vi "save_temperature_and_pressure_to_excel.vi"() -> ()   [LabVIEW 2019]
uses:
  <vilib>/Utility/NIReport.llb/Report Type.ctl
  <vilib>/Utility/NIReport.llb/Append Text Table to Report (wrap).vi
  <vilib>/Utility/NIReport.llb/NI_report.lvclass
  <vilib>/Utility/NIReport.llb/NI_ReportGenerationCore.lvlib
  <vilib>/Utility/NIReport.llb/Excel/NI_Excel.lvclass
panel:
  in  "report file path":path
  in  "stop":bool
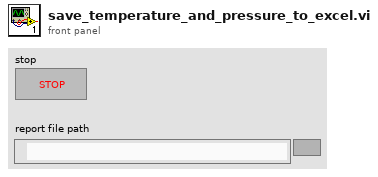
[diagram p1: front panel]
types:
  T1 = typedef "NI_ReportGenerationCore.lvlib/Report Type.ctl" = enum16{"HTML", "Word", "Excel"}
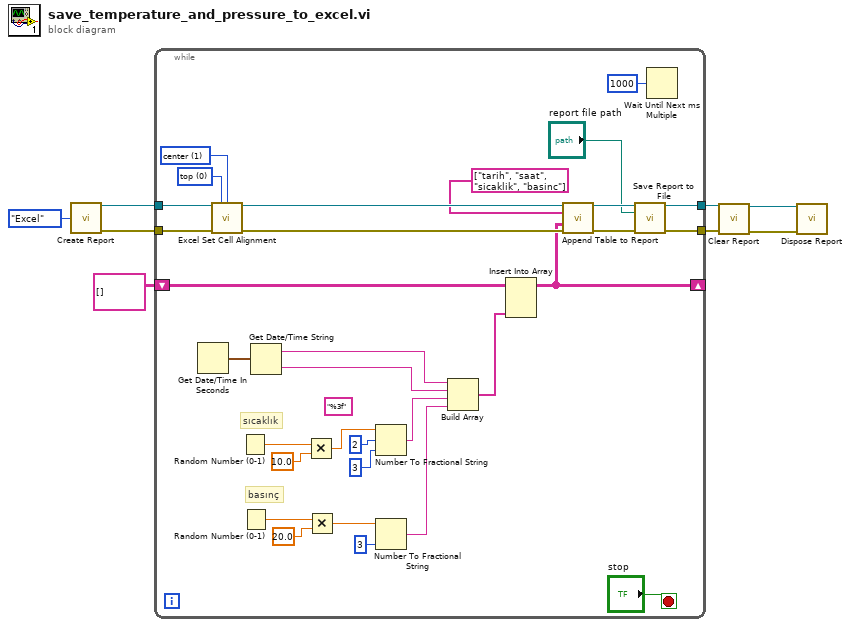
[diagram p0: block diagram]
diagram:
  n1 = call <vilib>:"Create Report.vi"("report type"=Report_Type."Excel") -> ("report out"=w7:refnum<class "NI_report.lvclass">, "error out"=w6:errorcluster)  [unwired: 13 in]
  n2 = while {
    tunnel: w7 -> [w35]
    tunnel: w6 -> [w34]
    tunnel: [w31] -> w4
    tunnel: [w30] -> w3
    shift-right: [w19] -> _
    shift-left: string[][] [] -> [w24]
    stop <- "stop" stop-if-true
    (unwired) "%3f" ("format string")
    w32 = 1 items=["left", "center", "right"] ("horizontal alignment (left)")
    w33 = 0 items=["top", "center", "bottom"] ("vertical alignment (top)")
    # "basınç"
    # "sıcaklık"
    n3 = Get Date/Time In Seconds() -> (seconds since 1Jan1904=w29:timestamp)
    n4 = call <vilib>:"Excel Set Cell Alignment.vi"("report in"=w35, "vertical alignment (top)"=w33, "horizontal alignment (left)"=w32, "error in (no error)"=w34) -> ("report out"=w23:refnum<class "NI_report.lvclass">, "error out"=w22:errorcluster)  [unwired: 10 in]
    n5 = Random Number (0-1)() -> (number: 0 to 1=w39:dbl)
    n6 = Random Number (0-1)() -> (number: 0 to 1=w37:dbl)
    n7 = Get Date/Time String(seconds (now)=w29) -> (date string=w28:string, time string=w27:string)  [unwired: 2 in]
    n8 = Multiply(x=w39, y=10.0) -> (x*y=w15:dbl)
    n9 = Multiply(x=w37, y=20.0) -> (x*y=w11:dbl)
    n10 = Number To Fractional String(number=w15, width (-)=i16 2, precision (6)=i16 3) -> (F-format string=w12:string)  [unwired: 1 in]
    n11 = Number To Fractional String(number=w11, precision (6)=i16 3) -> (F-format string=w10:string)  [unwired: 2 in]
    n12 = Build Array(w28, w27, w12, w10) -> (w25:string[])
    n13 = Insert Into Array(array=w24, new element=w25) -> (w19:string[][])  [unwired: 2 in]
    n14 = call-poly <vilib>:"Append Table to Report.vi"("report in"=w23, "column headers"=string[] ["tarih", "saat", "sicaklik", "basinc"], "text data"=w19, "error in (no error)"=w22) -> ("report out"=w21:refnum<class "NI_report.lvclass">, "error out"=w20:errorcluster)  [unwired: 8 in, 2 out]
    n15 = call-dynamic "Save Report to File.vi"("report in"=w21, "report file path"="report file path", "error in (no error)"=w20) -> ("report out"=w31:refnum<class "NI_report.lvclass">, "error out"=w30:errorcluster)  [unwired: 11 in]
    n16 = Wait Until Next ms Multiple(millisecond multiple=u32 1000) -> ()  [unwired: 1 out]
  }
  n17 = call-dynamic "Clear Report.vi"("report in"=w4, "error in (no error)"=w3) -> ("report out"=w2:refnum<class "NI_report.lvclass">, "error out"=w1:errorcluster)  [unwired: 12 in]
  n18 = call-dynamic "Dispose Report.vi"("report in"=w2, "error in (no error)"=w1) -> ()  [unwired: 13 in, 1 out]
